vi "Find-MTA-Doc-tag-in-vi-bin.vi"(8 "error in (no error)":errorcluster, 11 "Path":path=path "/user/pma/users/oddoa/LabVIEW-8.6/Projects/Vi-Documentation/prev/TestViProject/CMW Wrapper/My Main VI.vi") -> (0 "error out":errorcluster, 2 "found??":bool)   [LabVIEW 2014]
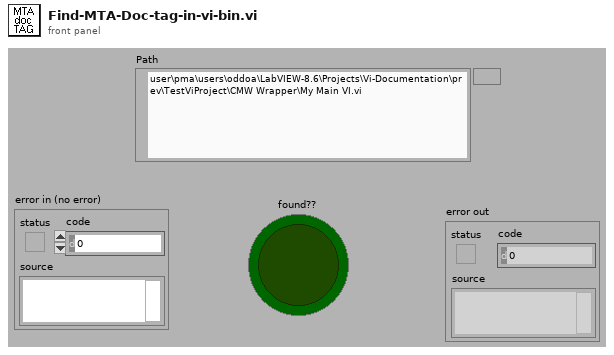
[diagram p1: front panel]
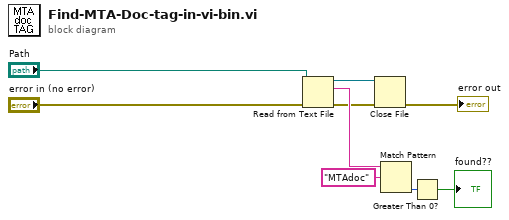
[diagram p0: block diagram]
diagram:
  n1 = Read from Text File(file (use dialog)="Path", error in="error in (no error)") -> (refnum out=w4:refnum<file>, text=w8:string, error out=w3:errorcluster)  [unwired: 3 out]
  n2 = Close File(refnum=w4, error in=w3) -> (error out=→"error out":errorcluster)  [unwired: 1 out]
  n3 = Match Pattern(string=w8, regular expression="MTAdoc") -> (offset past match=w6:i32)  [unwired: 4 out]
  n4 = Greater Than 0?(x=w6) -> (x > 0?=→"found??":bool)
